vi "SV TDMS Write Spectrum (Waterfall).vi"(0 "tdms file":refnum<k34>, 5 "group name in":string="Spectrum_Waterfall", 7 "channel names in":string[](array[string]), 9 "waterfall graph data":T2, 11 "error in":errorcluster, 12 "Z info":T1={"Z-axis label"="Z", "Z-unit string"=""}, 13 "spectrum info":T3 {"x-axis units" items=["Time (s)"=0, "Frequency-CB (Hz)"=1, "Frequency-CPB (Hz)"=1248, "Frequency-Arbitrary (Hz)"=2357, "Quefrency (s)"=2, "Revolutions (rev)"=3, "Order"=4, "Speed (RPM)"=11, "Speed (rad/s)"=21, "Index"=65535]; "weighting filter" items=["Linear", "A-weighting", "B-weighting", "C-weighting", "ITU-R 468-4", "Dolby", "CCITT", "C-message", "Wb", "Wc", "Wd", "We", "Wf", "Wh", "Wj", "Wk", "Wm", "AES17 20 kHz lowpass", "AES17 40 kHz lowpass", "AES17 20 kHz highpass", "AES17 40 kHz highpass"]; "dB reference [EU]" format="%.2f"; "engineering units" items=["custom..."=0, "V"=1, "A"=21, "C"=30, "pC"=31, "s"=32, "-"=29, "Pa"=2, "N"=20, "g"=3, "m/s^2"=4, "m/s"=5, "m"=6, "mm/s"=12, "mm"=13, "micron/s"=14, "micron"=15, "in/s^2"=7, "in/s"=8, "in"=9, "mil/s"=10, "mil"=11, "rad/s^2"=16, "rad/s"=17, "rad"=18, "deg/s^2"=26, "deg/s"=27, "deg"=28, "RPM"=22, "cycle/s^2"=23, "Hz"=24, "cycle"=25, "strain"=19]; "spectral info"."window" items=["None "=0, "Hanning"=1, "Hamming"=2, "Blackman-Harris"=3, "Exact Blackman"=4, "Blackman"=5, "Flat Top"=6, "4 Term B-Harris "=7, "7 Term B-Harris"=8, "Low Sidelobe"=9, "Force - Exponential"=10, "Gaussian"=62]}) -> (4 "tdms file out":refnum<k34>, 6 "group name out":string, 8 "channel names out":string[](array[string]), 15 "error out":errorcluster)   [LabVIEW 2017]
doc: "Writes data to the specified .tdms file in a format specific to the polymorphic instance. Wire data to the <B>scaled signal [EU]</B> input to determine the polymorphic instance to use or manually select the instance."
uses:
  <vilib>/addons/_NISVFA/_Shared subVIs/Controls/svc_Spectrum Info.ctl
  <vilib>/addons/_NISVFA/_Shared subVIs/Controls/svc_X-Axis Units.ctl
  <vilib>/addons/_NISVFA/_Shared subVIs/Controls/svc_Spectrum Type.ctl
  <vilib>/addons/_NISVFA/_Shared subVIs/Controls/svc_Engineering Units Text Ring.ctl
  <vilib>/addons/_NISVFA/_Shared subVIs/Controls/svc_Weighting Filter Text Ring.ctl
  <vilib>/addons/_NISVFA/_Shared subVIs/Controls/svc_Complimentary Spectrum Units.ctl
  <vilib>/addons/_NISVFA/_Shared subVIs/Controls/NI Channel Properties.ctl
  <vilib>/addons/_NISVFA/_Shared subVIs/Controls/LV Datatypes.ctl
  <vilib>/addons/_NISVFA/_Shared subVIs/Controls/NI Spectrum Component.ctl
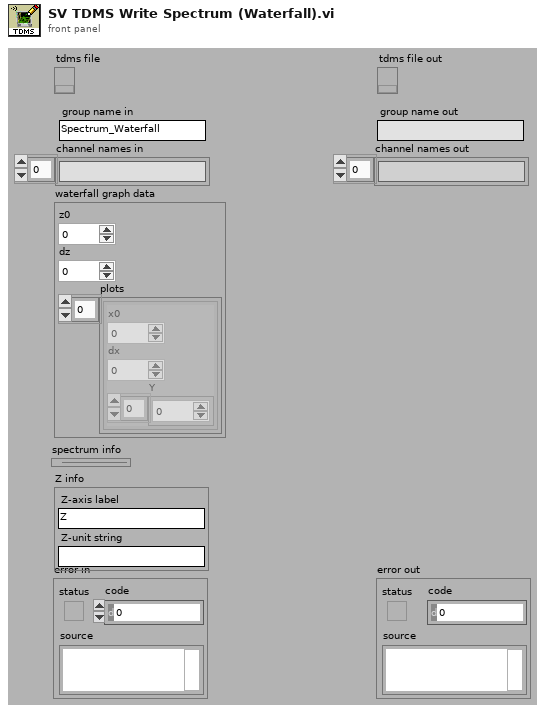
[diagram p1: front panel]
types:
  T1 = cluster{"Z-axis label":string, "Z-unit string":string}
  T2 = cluster{"z0":dbl, "dz":dbl, "plots":cluster{"x0":dbl, "dx":dbl, "Y":dbl[]}[]}
  T3 = typedef "svc_Spectrum Info.ctl" = cluster{"channel name":string, "description":string, "x-axis units":T4, "spectral info":cluster{"spectrum type":T5, "linear/dB":enum16{"linear", "dB"}, "window":u16, "window size":i32, "FFT size":i32}, "engineering units":T6, "custom label":string, "dB reference [EU]":dbl, "peak units":enum16{"rms", "peak", "peak-peak"}, "weighting filter":T7, "spectral density?":bool, "unit label":string, "spectrum skewed?":bool, "complimentary spectrum units":T8}
  T4 = typedef "svc_X-Axis Units.ctl" = u16
  T5 = typedef "svc_Spectrum Type.ctl" = enum16{"FFT Spectrum [complex]", "Amplitude [Magnitude]", "Power [Magnitude^2]", "Cross Spectrum [complex]", "Frequency Response [Complex]"}
  T6 = typedef "svc_Engineering Units Text Ring.ctl" = u16
  T7 = typedef "svc_Weighting Filter Text Ring.ctl" = u16
  T8 = typedef "svc_Complimentary Spectrum Units.ctl" = enum16{"none", "radians", "degrees", "cycles", "imaginary"}
  T9 = typedef "NI Spectrum Component.ctl" = u16
  T10 = typedef "LV Datatypes.ctl" = i32
  T11 = typedef "NI Channel Properties.ctl" = u16
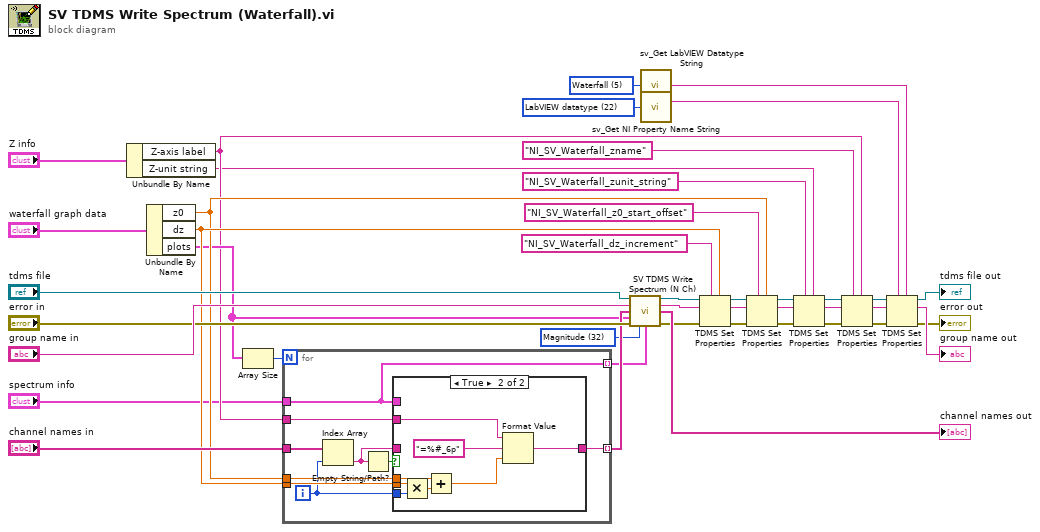
[diagram p0: block diagram]
diagram:
  w2 = T9 32 items=["Magnitude"=32, "Phase"=33, "Real"=34, "Imaginary"=35, "Coherence"=36, "Unknown"=99] ("spectrum component")
  w13 = T10 5 items=["String: abc"=-2, "Boolean: True or False"=-1, "Scalar: y"=0, "Array: Y"=1, "Waveform: t0, dt, Y, variant"=2, "Cluster: x0, dx, Y"=3, "Cluster: X, Y"=4, "Waterfall"=5, "Colormap"=6] ("LabVIEW datatype")
  w12 = T11 22 items=["Channel name", "Channel description", "Y-axis label", "Y-axis unit string", "X-axis label", "X-axis unit string", "x0", "dx", "Number of samples", "X channel", "Filter settled", "dB reference", "Window", "Window parameter", "Window size", "FFT size", "Peak units", "Spectrum type", "Magnitude scale", "Spectral density", "Sensor sensitivity (mV/EU)", "X-axis domain", "LabVIEW datatype"] ("property")
  n1 = Unbundle By Name("Z info") -> ("Z-axis label"=w15:string, "Z-unit string"=w14:string)
  n2 = Unbundle By Name("waterfall graph data") -> ("z0"=w23:dbl, "dz"=w24:dbl, "plots"=w21:cluster{"x0":dbl, "dx":dbl, "Y":dbl[]}[])
  n3 = Array Size(array=w21) -> (size(s)=w22:i32)
  n4 = for {
    N: w22 -> [_]
    tunnel: "channel names in" -> [w47]
    tunnel: "spectrum info" -> [w45]
    tunnel: [w51] -> w25 mode=indexing
    tunnel: w24 -> [w50]
    tunnel: w23 -> [w49]
    tunnel: [w45] -> w3 mode=indexing
    tunnel: w15 -> [w44]
    i -> [w46]
    n5 = Index Array(array=w47, index=w46) -> (element=w48:string)
    n6 = Empty String/Path?(string/path=w48) -> (empty?=w52:bool)
    n7 = case shown="True" w52 {
      tunnel: w45 -> [_ _]
      tunnel: w48 -> [w53 _]
      tunnel: [w53 w54] -> w51
      tunnel: w46 -> [_ w61]
      tunnel: w50 -> [_ w60]
      tunnel: w49 -> [_ w58]
      tunnel: w44 -> [_ w55]
      frame False {
      }
      frame True {
        n8 = Multiply(x=w60, y=w61) -> (x*y=w59:dbl)
        n9 = Add(x=w58, y=w59) -> (x+y=w57:dbl)
        n10 = Format Value(string ("")=w55, format string="=%#_6p", value (0)=w57) -> (output string=w54:string)
      }
    }
  }
  n11 = call <vilib>:"SV TDMS Write Spectrum (N Ch).vi"("tdms file"="tdms file", "group name in"="group name in", "channel names in"=w25, "spectra"=w21, "error in"="error in", "component"=w2, "spectra info"=w3) -> ("tdms file out"=w35:refnum<k34>, "group name out"=w36:string, "channel names out"=→"channel names out":string[], "error out"=w37:errorcluster)  [unwired: 5 in]
  n12 = call <vilib>:"sv_Get LabVIEW Datatype String.vi"("LabVIEW datatype"=w13) -> ("datatype string"=w5:string)  [unwired: 4 in]
  n13 = call <vilib>:"sv_Get NI Property Name String.vi"("property"=w12) -> ("TDMS property name"=w6:string)  [unwired: 13 in, 1 out]
  n14 = TDMS Set Properties(5:w24, 7:"NI_SV_Waterfall_dz_increment" ("channel name"), 8:w37, 10:w36, 11:w35) -> (0:w28:errorcluster, 2:w29:string, 3:w30:refnum<k34>)  [unwired: 1 in, 1 out]
  n15 = TDMS Set Properties(5:w23, 7:"NI_SV_Waterfall_z0_start_offset" ("channel name"), 8:w28, 10:w29, 11:w30) -> (0:w38:errorcluster, 2:w39:string, 3:w40:refnum<k34>)  [unwired: 1 in, 1 out]
  n16 = TDMS Set Properties(5:w14, 7:"NI_SV_Waterfall_zunit_string" ("channel name"), 8:w38, 10:w39, 11:w40) -> (0:w20:errorcluster, 2:w19:string, 3:w18:refnum<k34>)  [unwired: 1 in, 1 out]
  n17 = TDMS Set Properties(5:w15, 7:"NI_SV_Waterfall_zname" ("channel name"), 8:w20, 10:w19, 11:w18) -> (0:w11:errorcluster, 2:w10:string, 3:w9:refnum<k34>)  [unwired: 1 in, 1 out]
  n18 = TDMS Set Properties(5:w5, 7:w6, 8:w11, 10:w10, 11:w9) -> (0:→"error out":errorcluster, 2:→"group name out":string, 3:→"tdms file out":refnum<k34>)  [unwired: 1 in, 1 out]
